vi "Specific Path to Common Path.vi"(10 "specific path":path) -> (2 "common path":string)   [LabVIEW 2020, in "NI_LVConfig.lvlib"]
uses:
  NI_LVConfig.lvlib
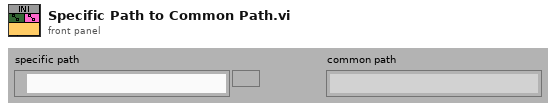
[diagram p1: front panel]
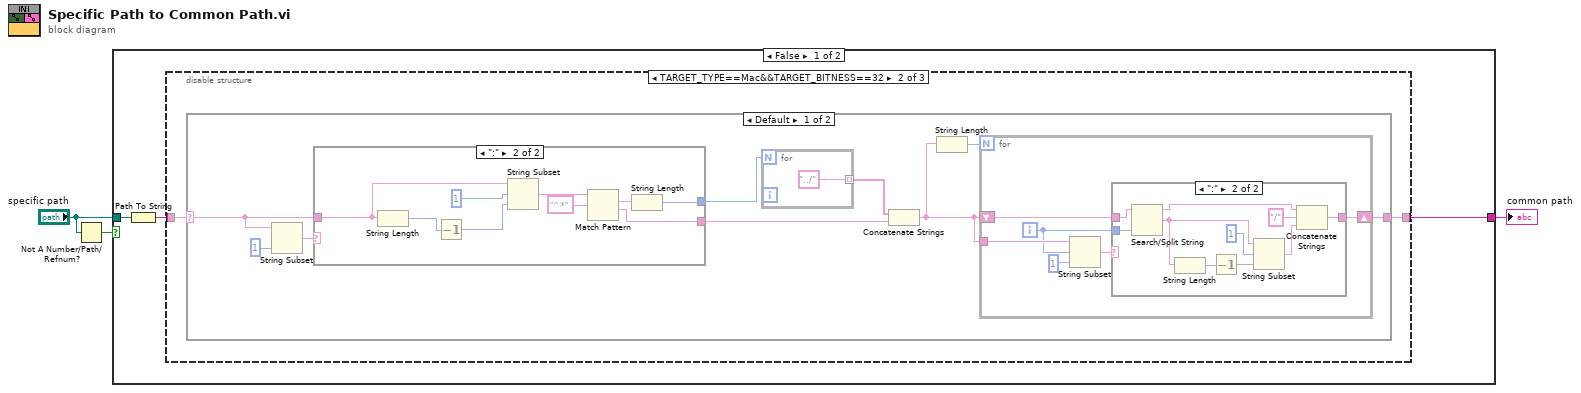
[diagram p0: block diagram]
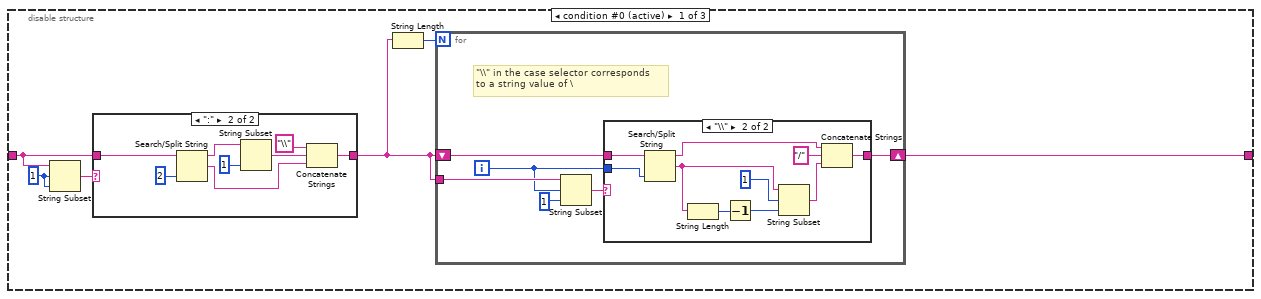
[diagram p2: hidden frame]
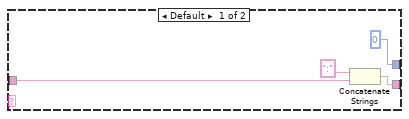
[diagram p6: hidden frame]
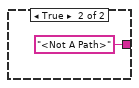
[diagram p9: hidden frame]
diagram:
  n1 = Not A Number/Path/Refnum?(number/path/refnum="specific path") -> (NaN/Path/Refnum?=w3:bool)
  n2 = case shown="False" w3 {
    tunnel: "specific path" -> [w6 _]
    tunnel: [w4 "<Not A Path>" ("string")] -> w1
    frame False {
      n3 = Path To String(path=w6) -> (string=w5:string)
      n4 = disable-structure "Conditional Disable Structure" shown="TARGET_TYPE==Mac&&TARGET_BITNESS==32" {
        disable-tunnel: w5 -> [w8 w39 w82]
        disable-tunnel: [w7 w40 w82] -> w4
        frame condition #0 (active) {
          w12 = 1 ("length")
          n5 = String Subset(string=w8, offset (0)=w12, length (rest)=w12) -> (substring=w9:string)
          n6 = case shown="\":\"" w9 {
            tunnel: w8 -> [w30 w38]
            tunnel: [w30 w34] -> w10
            frame Default {
            }
            frame ":" {
              n7 = Search/Split String(string=w38, offset (0)=2) -> (substring before match=w36:string, match + rest of string=w35:string)  [unwired: 2 out]
              n8 = String Subset(string=w36, length (rest)=1 ("offset (0)")) -> (substring=w32:string)  [unwired: 1 out]
              n9 = Concatenate Strings("\\", w32, w35) -> (w34:string)
            }
          }
          n10 = String Length(string=w10) -> (length=w11:i32)
          n11 = for {
            N: w11 -> [_]
            tunnel: w10 -> [w16]
            shift-right: [w17] -> w7
            shift-left: w10 -> [w18]
            i -> [w15]
            # "\"\\\\\" in the case selector corresponds\nto a string value of \\"
            n12 = String Subset(string=w16, offset (0)=w15, length (rest)=1 ("length")) -> (substring=w13:string)
            n13 = case shown="\"\\\\\"" w13 {
              tunnel: w18 -> [w19 w29]
              tunnel: w15 -> [_ w21]
              tunnel: [w19 w27] -> w17
              frame Default {
              }
              frame "\\" {
                n14 = Search/Split String(string=w29, offset (0)=w21) -> (substring before match=w28:string, match + rest of string=w25:string)  [unwired: 2 out]
                n15 = String Length(string=w25) -> (length=w24:i32)
                n16 = Decrement(x=w24) -> (x-1=w23:i32)
                n17 = String Subset(string=w25, offset (0)=1, length (rest)=w23) -> (substring=w20:string)
                n18 = Concatenate Strings(w28, "/" ("x"), w20) -> (w27:string)
              }
            }
          }
        }
        frame condition #1 {
          n19 = case shown="Default" w39 {
            selector: w39 -> [w42 w81]
            tunnel: [w43 w81] -> w40
            frame Default {
              n20 = String Subset(string=w42, length (rest)=1 ("length")) -> (substring=w41:string)  [unwired: 1 out]
              n21 = case shown="\":\"" w41 {
                tunnel: w42 -> [w71 w72]
                tunnel: [w69 w75] -> w47
                tunnel: [0 w74] -> w48
                frame Default {
                  n22 = Concatenate Strings(":", w71) -> (w69:string)
                }
                frame ":" {
                  n23 = String Length(string=w72) -> (length=w80:i32)
                  n24 = Decrement(x=w80) -> (x-1=w79:i32)
                  n25 = String Subset(string=w72, offset (0)=1 ("length"), length (rest)=w79) -> (substring=w73:string)
                  n26 = Match Pattern(string=w73, regular expression="^:*") -> (match substring=w76:string, after substring=w75:string)  [unwired: 3 out]
                  n27 = String Length(string=w76) -> (length=w74:i32)
                }
              }
              n28 = for {
                N: w48 -> [_]
                tunnel: ["../"] -> w46 mode=indexing
              }
              n29 = Concatenate Strings(w46, w47) -> (w44:string)
              n30 = String Length(string=w44) -> (length=w45:i32)
              n31 = for {
                N: w45 -> [_]
                tunnel: w44 -> [w53]
                shift-right: [w54] -> w43
                shift-left: w44 -> [w55]
                i -> [w52]
                n32 = String Subset(string=w53, offset (0)=w52, length (rest)=1 ("length")) -> (substring=w50:string)
                n33 = case shown="\":\"" w50 {
                  tunnel: w55 -> [w56 w66]
                  tunnel: w52 -> [_ w58]
                  tunnel: [w56 w64] -> w54
                  frame Default {
                  }
                  frame ":" {
                    n34 = Search/Split String(string=w66, offset (0)=w58) -> (substring before match=w65:string, match + rest of string=w62:string)  [unwired: 2 out]
                    n35 = String Length(string=w62) -> (length=w61:i32)
                    n36 = Decrement(x=w61) -> (x-1=w60:i32)
                    n37 = String Subset(string=w62, offset (0)=1, length (rest)=w60) -> (substring=w57:string)
                    n38 = Concatenate Strings(w65, "/" ("x"), w57) -> (w64:string)
                  }
                }
              }
            }
            frame "" {
            }
          }
        }
        frame condition #2 {
        }
      }
    }
    frame True {
    }
  }
  "common path" <- w1
